vi "Go_to_posn_tl.vi"(1 "Channel Name":string, 3 "error in (no error)":errorcluster, 4 "Position":i32=1 min=1 max=16, 5 "Port Name":string, 6 "Valve Number":i32 max=9 step=1) -> (0 "error out":errorcluster)   [LabVIEW 2010]
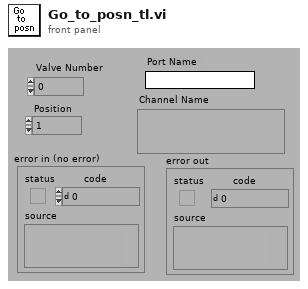
[diagram p1: front panel]
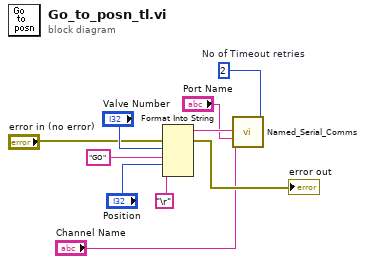
[diagram p0: block diagram]
diagram:
  w3 = 2  # No of Timeout retries
  n1 = Format Into String(error in="error in (no error)", "Valve Number", "GO", "Position", "\r") -> (resulting string=w7:string, error out=→"error out":errorcluster)  [unwired: 2 in]
  n2 = call "Named_Serial_Comms.vi"("Channel Name"="Channel Name", "Write String"=w7, "!Timeout retries"=w3, "Port Name"="Port Name") -> ()  [unwired: 5 in, 7 out]
